vi "Creating JSON Data.vi"() -> ()   [LabVIEW 2015]
uses:
  <vilib>/NI/JSON Support for LabVIEW/JSON Data Classes/JSON String/New JSON String.vi
  <vilib>/NI/JSON Support for LabVIEW/JSON Data Classes/JSON Numeric/New JSON Numeric.vi
  <vilib>/NI/JSON Support for LabVIEW/JSON Data Classes/JSON Boolean/New JSON Boolean.vi
  <vilib>/NI/JSON Support for LabVIEW/JSON Data Classes/JSON Datatype/New JSON Null.vi
  <vilib>/NI/JSON Support for LabVIEW/JSON Data Classes/JSON Array/New JSON Array (String).vi
  <vilib>/NI/JSON Support for LabVIEW/JSON Data Classes/JSON Array/New JSON Array (Numeric).vi
  <vilib>/NI/JSON Support for LabVIEW/JSON Data Classes/JSON Array/New JSON Array (Boolean).vi
  <vilib>/NI/JSON Support for LabVIEW/JSON Data Classes/JSON Array/New JSON Array (Empty).vi
  <vilib>/NI/JSON Support for LabVIEW/JSON Data Classes/JSON Object/New JSON Object (Single Numeric).vi
  <vilib>/NI/JSON Support for LabVIEW/JSON Data Classes/JSON Array/New JSON Array (JSON Data).vi
  <vilib>/NI/JSON Support for LabVIEW/JSON Data Classes/JSON Object/New JSON Object (Empty).vi
  <vilib>/NI/JSON Support for LabVIEW/JSON Data Classes/JSON Object/New JSON Object (Single String).vi
  <vilib>/NI/JSON Support for LabVIEW/JSON Data Classes/JSON Object/New JSON Object (Multi).vi
  <vilib>/NI/JSON Support for LabVIEW/JSON Data Classes/JSON Datatype/JSON Null.lvclass
  <vilib>/NI/JSON Support for LabVIEW/JSON Data Classes/JSON Object/JSON Object.lvclass
  <vilib>/NI/JSON Support for LabVIEW/JSON Data Classes/JSON Array/JSON Array.lvclass
  <vilib>/NI/JSON Support for LabVIEW/JSON Data Classes/JSON String/JSON String.lvclass
  <vilib>/NI/JSON Support for LabVIEW/JSON Data Classes/JSON Numeric/JSON Numeric.lvclass
  <vilib>/NI/JSON Support for LabVIEW/JSON Data Classes/JSON Boolean/JSON Boolean.lvclass
  <vilib>/NI/JSON Support for LabVIEW/JSON Data Classes/JSON Helper/JSON Helper.lvclass
panel:
  out "JSON Array of JSON Instances":string
  out "Empty JSON Object":string
  out "JSON Object with Single String Parameter":string
  out "JSON Object with Multiple JSON Parameters":string
  out "JSON Arry of Strings":string
  out "JSON Array of Numerics":string
  out "JSON Array of Booleans":string
  out "Empty JSON Array":string
  out "JSON Boolean":string
  out "JSON Null":string
  out "JSON Numeric":string
  out "JSON String":string
  # "Creating a JSON Null Value"
  # "Creating JSON Literal Values"
  # "Creating JSON Arrays"
  # "Creating JSON Objects"
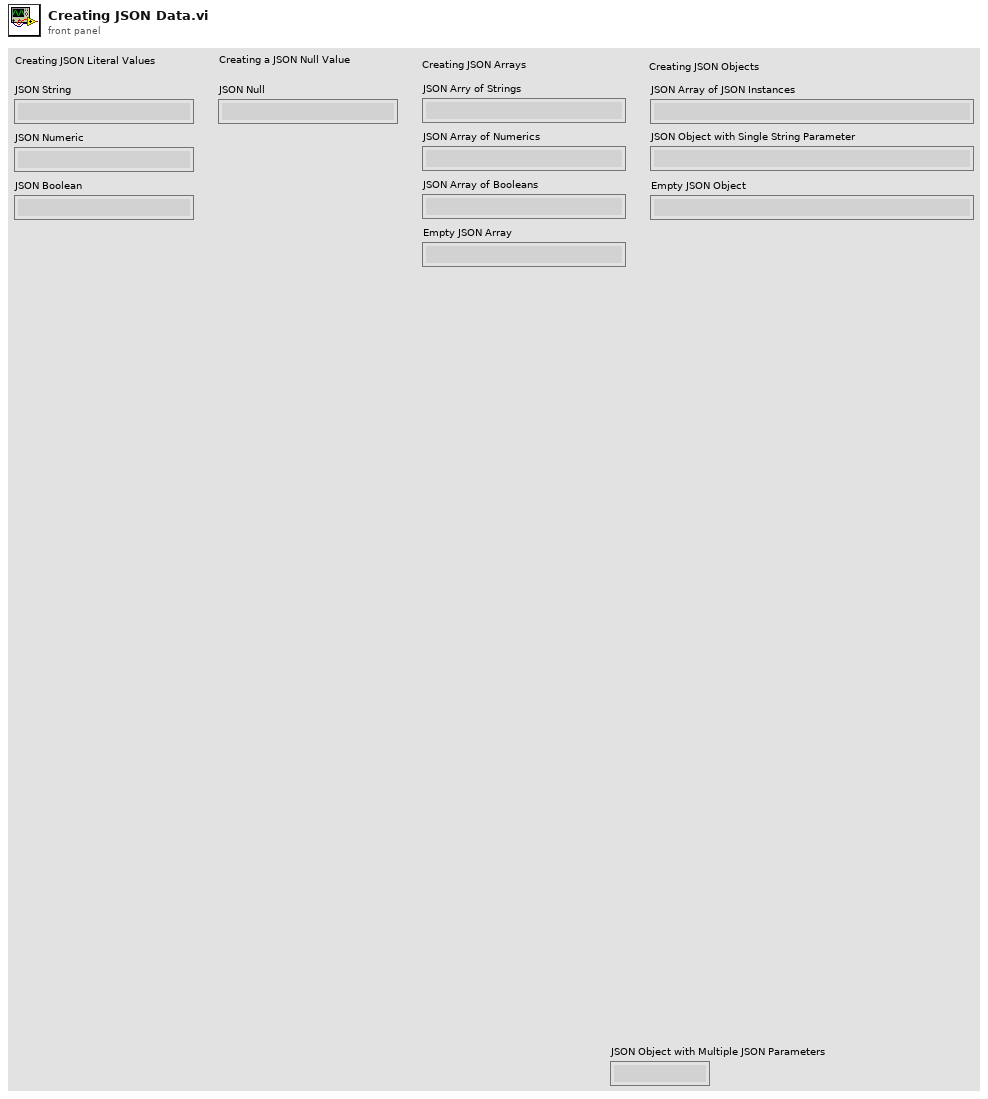
[diagram p1: front panel]
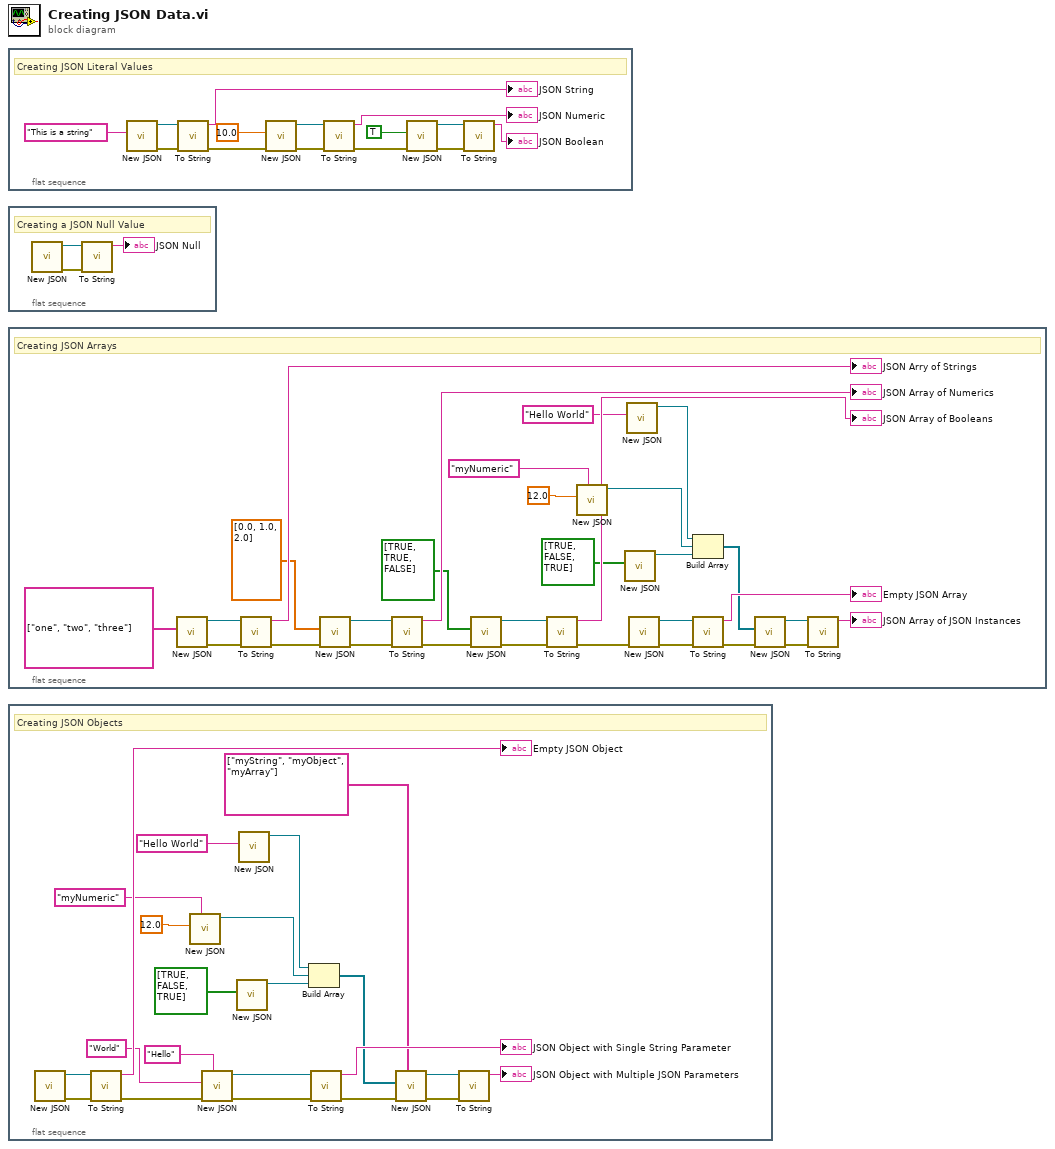
[diagram p0: block diagram]
diagram:
  n1 = flat-sequence {
    frame #0 {
      # "Creating JSON Literal Values"
      n2 = call-poly <vilib>:"New JSON.vi"("value"="This is a string") -> ("error out"=w3:errorcluster, "JSON String out"=w11:refnum<class "JSON String.lvclass">)  [unwired: 9 in]
      n3 = call-dynamic "To String.vi"("error in (no error)"=w3, "JSON String in"=w11) -> ("error out"=w2:errorcluster, "String"=→"JSON String":string)  [unwired: 8 in]
      n4 = call-poly <vilib>:"New JSON.vi"("error in (no error)"=w2, "value"=10.0) -> ("error out"=w8:errorcluster, "JSON String out"=w7:refnum<class "JSON Numeric.lvclass">)  [unwired: 8 in]
      n5 = call-dynamic "To String.vi"("error in (no error)"=w8, "JSON Numeric in"=w7) -> ("error out"=w1:errorcluster, "String"=→"JSON Numeric":string)  [unwired: 8 in]
      n6 = call-poly <vilib>:"New JSON.vi"("error in (no error)"=w1, "value"=TRUE) -> ("error out"=w4:errorcluster, "JSON String out"=w5:refnum<class "JSON Boolean.lvclass">)  [unwired: 8 in]
      n7 = call-dynamic "To String.vi"("error in (no error)"=w4, "JSON Boolean in"=w5) -> ("String"=→"JSON Boolean":string)  [unwired: 8 in, 1 out]
    }
  }
  n8 = flat-sequence {
    frame #0 {
      # "Creating a JSON Null Value"
      n9 = call-poly <vilib>:"New JSON.vi"() -> ("error out"=w17:errorcluster, "JSON Null out"=w16:refnum<class "JSON Null.lvclass">)  [unwired: 10 in]
      n10 = call-dynamic "To String.vi"("error in (no error)"=w17, "JSON Datatype in"=w16) -> ("String"=→"JSON Null":string)  [unwired: 8 in, 1 out]
    }
  }
  n11 = flat-sequence {
    frame #0 {
      # "Creating JSON Arrays"
      n12 = call-poly <vilib>:"New JSON.vi"("String Array"=string[] ["one", "two", "three"]) -> ("error out"=w43:errorcluster, "JSON Array out"=w27:refnum<class "JSON Array.lvclass">)  [unwired: 9 in]
      n13 = call-dynamic "To String.vi"("error in (no error)"=w43, "JSON Array in"=w27) -> ("error out"=w36:errorcluster, "String"=→"JSON Arry of Strings":string)  [unwired: 8 in]
      n14 = call-poly <vilib>:"New JSON.vi"("error in (no error)"=w36, "Numeric Array"=dbl[] [0.0, 1.0, 2.0]) -> ("error out"=w42:errorcluster, "JSON Array out"=w30:refnum<class "JSON Array.lvclass">)  [unwired: 8 in]
      n15 = call-dynamic "To String.vi"("error in (no error)"=w42, "JSON Array in"=w30) -> ("error out"=w35:errorcluster, "String"=→"JSON Array of Numerics":string)  [unwired: 8 in]
      n16 = call-poly <vilib>:"New JSON.vi"("error in (no error)"=w35, "Boolean Array"=bool[] [TRUE, TRUE, FALSE]) -> ("error out"=w41:errorcluster, "JSON Array out"=w29:refnum<class "JSON Array.lvclass">)  [unwired: 8 in]
      n17 = call-dynamic "To String.vi"("error in (no error)"=w41, "JSON Array in"=w29) -> ("error out"=w34:errorcluster, "String"=→"JSON Array of Booleans":string)  [unwired: 8 in]
      n18 = call-poly <vilib>:"New JSON.vi"("key"="myNumeric", "value"=12.0) -> ("JSON Object out"=w20:refnum<class "JSON Object.lvclass">)  [unwired: 8 in, 1 out]
      n19 = call-poly <vilib>:"New JSON.vi"("Boolean Array"=bool[] [TRUE, FALSE, TRUE]) -> ("JSON Array out"=w19:refnum<class "JSON Array.lvclass">)  [unwired: 9 in, 1 out]
      n20 = call-poly <vilib>:"New JSON.vi"("value"="Hello World") -> ("JSON String out"=w23:refnum<class "JSON String.lvclass">)  [unwired: 9 in, 1 out]
      n21 = call-poly <vilib>:"New JSON.vi"("error in (no error)"=w34) -> ("error out"=w40:errorcluster, "JSON Array out"=w28:refnum<class "JSON Array.lvclass">)  [unwired: 9 in]
      n22 = Build Array(w23, w20, w19) -> (w25:refnum<class "JSON Null.lvclass">[])
      n23 = call-dynamic "To String.vi"("error in (no error)"=w40, "JSON Array in"=w28) -> ("error out"=w26:errorcluster, "String"=→"Empty JSON Array":string)  [unwired: 8 in]
      n24 = call-poly <vilib>:"New JSON.vi"("error in (no error)"=w26, "JSON Datatypes"=w25) -> ("error out"=w31:errorcluster, "JSON Array out"=w32:refnum<class "JSON Array.lvclass">)  [unwired: 8 in]
      n25 = call-dynamic "To String.vi"("error in (no error)"=w31, "JSON Array in"=w32) -> ("String"=→"JSON Array of JSON Instances":string)  [unwired: 8 in, 1 out]
    }
  }
  n26 = flat-sequence {
    frame #0 {
      # "Creating JSON Objects"
      n27 = call-poly <vilib>:"New JSON.vi"() -> ("error out"=w63:errorcluster, "JSON Object out"=w66:refnum<class "JSON Object.lvclass">)  [unwired: 10 in]
      n28 = call-dynamic "To String.vi"("error in (no error)"=w63, "JSON Object in"=w66) -> ("error out"=w62:errorcluster, "String"=→"Empty JSON Object":string)  [unwired: 8 in]
      n29 = call-poly <vilib>:"New JSON.vi"("key"="myNumeric", "value"=12.0) -> ("JSON Object out"=w55:refnum<class "JSON Object.lvclass">)  [unwired: 8 in, 1 out]
      n30 = call-poly <vilib>:"New JSON.vi"("key"="Hello", "error in (no error)"=w62, "value"="World") -> ("error out"=w60:errorcluster, "JSON Object out"=w65:refnum<class "JSON Object.lvclass">)  [unwired: 7 in]
      n31 = call-poly <vilib>:"New JSON.vi"("Boolean Array"=bool[] [TRUE, FALSE, TRUE]) -> ("JSON Array out"=w56:refnum<class "JSON Array.lvclass">)  [unwired: 9 in, 1 out]
      n32 = call-poly <vilib>:"New JSON.vi"("value"="Hello World") -> ("JSON String out"=w52:refnum<class "JSON String.lvclass">)  [unwired: 9 in, 1 out]
      n33 = Build Array(w52, w55, w56) -> (w50:refnum<class "JSON Null.lvclass">[])
      n34 = call-dynamic "To String.vi"("error in (no error)"=w60, "JSON Object in"=w65) -> ("error out"=w48:errorcluster, "String"=→"JSON Object with Single String Parameter":string)  [unwired: 8 in]
      n35 = call-poly <vilib>:"New JSON.vi"("keys"=string[] ["myString", "myObject", "myArray"] ("key"), "error in (no error)"=w48, "values"=w50) -> ("error out"=w61:errorcluster, "JSON Object out"=w64:refnum<class "JSON Object.lvclass">)  [unwired: 7 in]
      n36 = call-dynamic "To String.vi"("error in (no error)"=w61, "JSON Object in"=w64) -> ("String"=→"JSON Object with Multiple JSON Parameters":string)  [unwired: 8 in, 1 out]
    }
  }
